vi "Command - Output State.vi"(0 "VISA Refnum in":refnum<visa-resource-name>, 5 "Channel":i32, 7 "State":bool=TRUE, 11 "Error In":errorcluster, 12 "Command Type":enum16{"Set", "Get"}(ring)) -> (4 "VISA Refnum out":refnum<visa-resource-name>, 6 "Read Buffer":string, 15 "Error Out":errorcluster)   [LabVIEW 2025]
panel:
  out "return count":u32
  out "Command":string
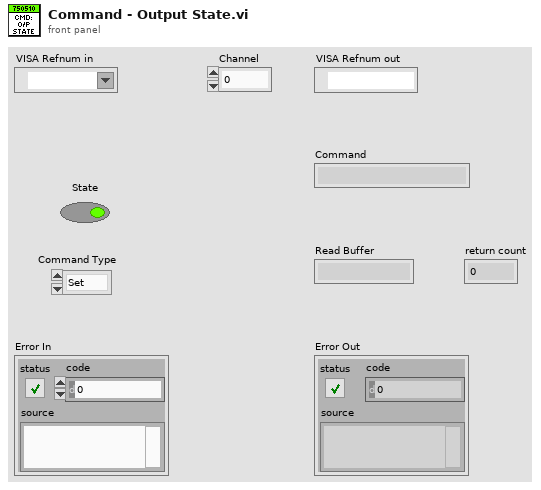
[diagram p1: front panel]
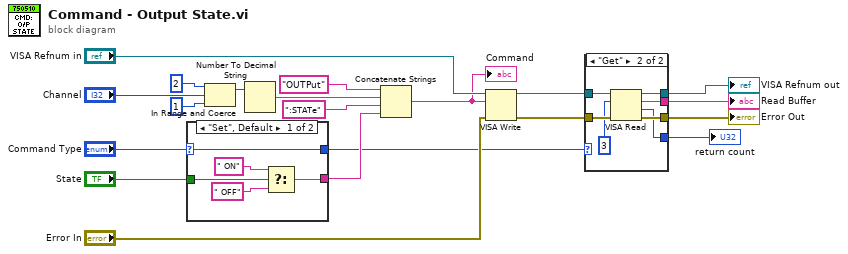
[diagram p0: block diagram]
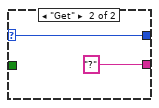
[diagram p2: hidden frame]
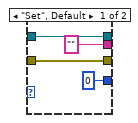
[diagram p3: hidden frame]
diagram:
  n1 = case shown="\"Set\", Default" "Command Type" {
    selector: "Command Type" -> [w21 w26]
    tunnel: [w23 "?" ("string")] -> w4
    tunnel: "State" -> [w22 _]
    tunnel: [w21 w26] -> w2
    frame "Set", Default {
      n2 = Select(t=" ON", s=w22, f=" OFF") -> (s? t:f=w23:string)
    }
    frame "Get" {
    }
  }
  n3 = In Range and Coerce(upper limit=2, x="Channel", lower limit=1) -> (coerced(x)=w9:i32)  [unwired: 1 out]
  n4 = Number To Decimal String(number=w9) -> (decimal integer string=w11:string)  [unwired: 1 in]
  n5 = Concatenate Strings("OUTPut", w11, ":STATe", w4) -> (w13:string)
  "Command" <- w13
  n6 = VISA Write(VISA resource name="VISA Refnum in", write buffer=w13, error in (no error)="Error In") -> (VISA resource name out=w15:refnum<visa-resource-name>, error out=w16:errorcluster)  [unwired: 1 out]
  n7 = case shown="\"Get\"" w2 {
    tunnel: w15 -> [w30 w38]
    tunnel: w16 -> [w31 w37]
    tunnel: [w31 w36] -> w17
    tunnel: [w30 w35] -> w18
    tunnel: ["" ("read buffer") w34] -> w19
    tunnel: [u32 0 ("return count") w32] -> w1
    frame "Set", Default {
    }
    frame "Get" {
      n8 = VISA Read(VISA resource name=w38, byte count=u32 3, error in (no error)=w37) -> (VISA resource name out=w35:refnum<visa-resource-name>, read buffer=w34:string, return count=w32:u32, error out=w36:errorcluster)
    }
  }
  "Read Buffer" <- w19
  "VISA Refnum out" <- w18
  "Error Out" <- w17
  "return count" <- w1
